vi "RANGE Auto Mode.vi"(5 "SLPM Error @ Zero (2,4,6)":dbl, 7 "SLPM Error @ Zero (1,3,5)":dbl, 8 "Error In":errorcluster, 10 "Meter 1,3,5":T1, 11 "Meter 2,4,6":T1) -> (0 "Error Out":errorcluster, 2 "Status":string, 3 "Meter Auto":T1)   [LabVIEW 2018]
uses:
  Drivers/Omega FMA-1600A Series Gas Flow Meter/Type Definitions/FMA1600A Data.ctl
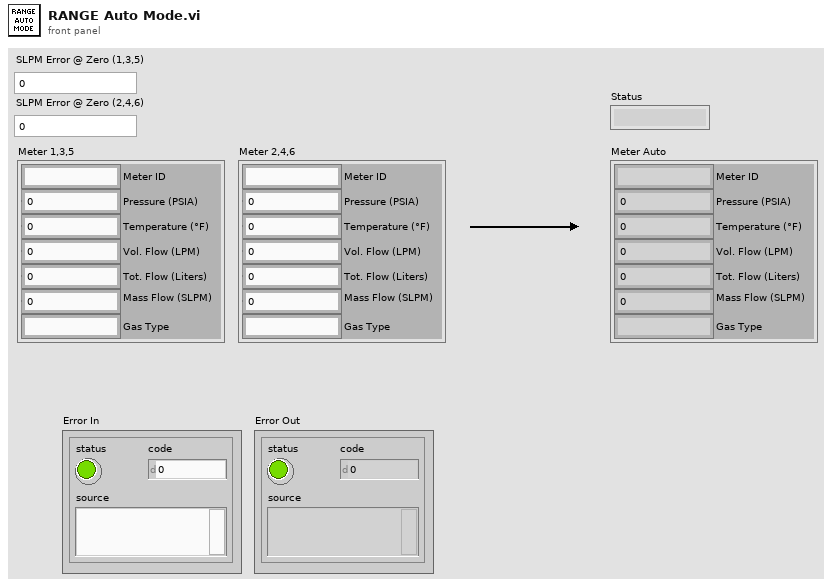
[diagram p1: front panel]
types:
  T1 = typedef "FMA1600A Data.ctl" = cluster{"Pressure (PSIA)":dbl, "Temperature (°F)":dbl, "Vol. Flow (LPM)":dbl, "Mass Flow (SLPM)":dbl, "Gas Type":string, "Tot. Flow (Liters)":dbl, "Meter ID":string}
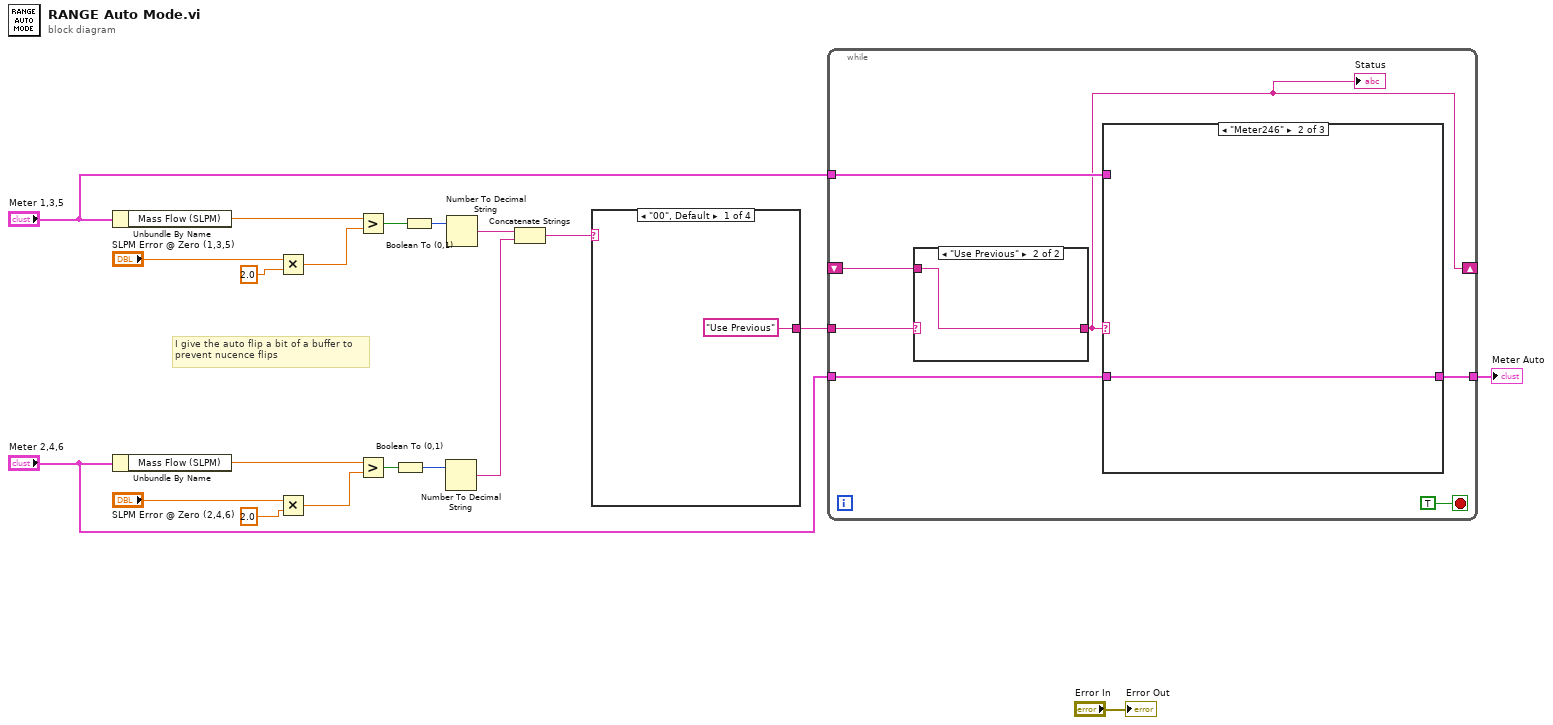
[diagram p0: block diagram]
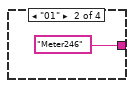
[diagram p2: hidden frame]
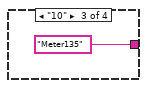
[diagram p3: hidden frame]
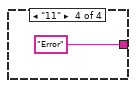
[diagram p4: hidden frame]
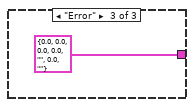
[diagram p7: hidden frame]
diagram:
  # "I give the auto flip a bit of a buffer to\nprevent nucence flips"
  n1 = Unbundle By Name("Meter 1,3,5") -> ("Mass Flow (SLPM)"=w14:dbl)
  n2 = Unbundle By Name("Meter 2,4,6") -> ("Mass Flow (SLPM)"=w12:dbl)
  n3 = Multiply(x="SLPM Error @ Zero (1,3,5)", y=2.0) -> (x*y=w13:dbl)
  n4 = Multiply(x="SLPM Error @ Zero (2,4,6)", y=2.0) -> (x*y=w11:dbl)
  n5 = Greater?(x=w14, y=w13) -> (0:w10:bool)
  n6 = Greater?(x=w12, y=w11) -> (0:w9:bool)
  n7 = Boolean To (0,1)(Boolean=w9) -> (0, 1=w7:i16)
  n8 = Boolean To (0,1)(Boolean=w10) -> (0, 1=w8:i16)
  n9 = Number To Decimal String(number=w7) -> (decimal integer string=w5:string)  [unwired: 1 in]
  n10 = Number To Decimal String(number=w8) -> (decimal integer string=w6:string)  [unwired: 1 in]
  n11 = Concatenate Strings(w6, w5) -> (w4:string)
  n12 = case shown="\"00\", Default" w4 {
    tunnel: ["Use Previous" "Meter246" "Meter135" "Error"] -> w1
    frame "00", Default {
    }
    frame "01" {
    }
    frame "10" {
    }
    frame "11" {
    }
  }
  n13 = while {
    tunnel: "Meter 1,3,5" -> [w31]
    tunnel: [w29] -> w3
    tunnel: "Meter 2,4,6" -> [w28]
    shift-right: [w25] -> _
    shift-left: _ -> [w27]
    tunnel: w1 -> [w26]
    stop <- TRUE stop-if-true
    n14 = case shown="\"Use Previous\"" w26 {
      selector: w26 -> [w32 _]
      tunnel: w27 -> [_ w33]
      tunnel: [w32 w33] -> w25
      frame Default {
      }
      frame "Use Previous" {
      }
    }
    "Status" <- w25
    n15 = case shown="\"Meter246\"" w25 {
      tunnel: w31 -> [w34 _ _]
      tunnel: [w34 w35 T1 {"Pressure (PSIA)"=0.0, "Temperature (°F)"=0.0, "Vol. Flow (LPM)"=0.0, "Mass Flow (SLPM)"=0.0, "Gas Type"="", "Tot. Flow (Liters)"=0.0, "Meter ID"=""} ("Meter 1,3,5")] -> w29
      tunnel: w28 -> [_ w35 _]
      frame "Meter135", Default {
      }
      frame "Meter246" {
      }
      frame "Error" {
      }
    }
  }
  "Meter Auto" <- w3
  "Error Out" <- "Error In"
